vi "PH_gentec_P-Link.set Default Settings.vi"(0 "i ref in":refnum<vi>, 5 "error in":errorcluster) -> (14 "i ref out":refnum<vi>, 19 "error out":errorcluster)   [LabVIEW 2014, in "PH_gentec_P-Link.lvlib"]
doc: "This VI sets Default Settings to wanted Device Settings at own attreibutes. This VI must be placed before the creation of the Proc Events in order to be able to overwrite these later by a Start GOG ..."
uses:
  PH_gentec_P-Link.lvlib
  PH_gentec_M-Link/PH_gentec_M-Link.lvlib
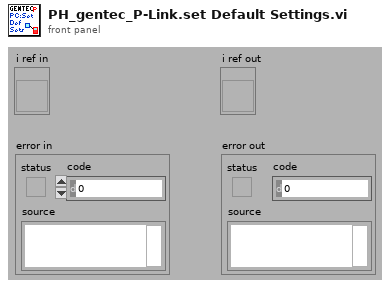
[diagram p1: front panel]
types:
  T1 = typedef "PH_gentec_P-Link.lvlib/PH_gentec_P-Link.i attribute.ctl" = cluster{"GUI References":cluster{"Wanted Head Settings":refnum<vi>, "Current Head Settings":refnum<vi>, "Set Auto Range":refnum<vi>, "Trigger Polarity":refnum<vi>, "Trigger Source":refnum<vi>, "Waveform Averages":refnum<vi>, "Continuous":refnum<vi>, "get one Value":refnum<vi>}, "Wanted Head Settings":T2, "Current Head Settings":T2}
  T2 = typedef "PH_gentec_P-Link.lvlib/PH_gentec_P-Link.Head Settings.ctl" = cluster{"Measurement Mode":T3, "Enable Anticipation":bool, "Set Auto Range":bool, "Block Signal":bool, "Set Head Attenuator":bool, "Enable SSE":bool, "Trigger Polarity":T4, "Trigger Source":T5, "Waveform Averages":T6, "Set Zero":i32, "Current":i32, "Start Data Flow":bool}
  T3 = typedef "gentec-M-Link - Driver.lvlib/gentec-M-Link.Measurement Mode.ctl" = u16
  T4 = typedef "gentec-M-Link - Driver.lvlib/gentec-M-Link.Trigger Polarity.ctl" = u16
  T5 = typedef "gentec-M-Link - Driver.lvlib/gentec-M-Link.Trigger Source.ctl" = u16
  T6 = typedef "gentec-M-Link - Driver.lvlib/gentec-M-Link.Waveform Averages.ctl" = u16
  T7 = typedef "PH_gentec_M-Link.lvlib/PH_gentec_M-Link.Head Settings.ctl" = cluster{"Measurement Mode":T8, "Enable Anticipation":bool, "Set Auto Range":bool, "Block Signal":bool, "Set Head Attenuator":bool, "Range":T9, "Enable SSE":bool, "Trigger Level [%]":dbl, "Trigger Polarity":T10, "Trigger Source":T11, "Waveform Averages":T12, "Wavelength [nm]":u16, "Set Zero":i32, "Current Measurement":i32, "Start Data Flow":bool}
  T8 = typedef "gentec-M-LINK.lvlib/gentec-M-Link.Measurement Mode.ctl" = u16
  T9 = typedef "gentec-M-LINK.lvlib/gentec-M-Link.Range.ctl" = u16
  T10 = typedef "gentec-M-LINK.lvlib/gentec-M-Link.Trigger Polarity.ctl" = u16
  T11 = typedef "gentec-M-LINK.lvlib/gentec-M-Link.Trigger Source.ctl" = u16
  T12 = typedef "gentec-M-LINK.lvlib/gentec-M-Link.Waveform Averages.ctl" = u16
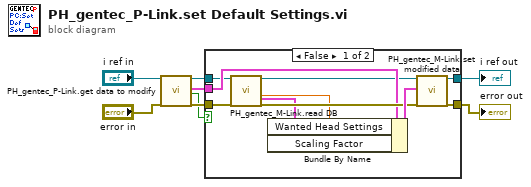
[diagram p0: block diagram]
diagram:
  n1 = call "PH_gentec_P-Link.get data to modify.vi"("i ref in"="i ref in", "error in (no error)"="error in") -> ("i ref out"=w6:refnum<vi>, "i attribute"=w4:T1, "timed out"=w3:bool, "error out"=w5:errorcluster)  [unwired: 14 in]
  n2 = case shown="False" w3 {
    tunnel: [w10 w19] -> w8
    tunnel: [w11 w20] -> w7
    tunnel: w5 -> [w17 w19]
    tunnel: w6 -> [w13 w20]
    tunnel: w4 -> [w15 _]
    frame False {
      n3 = call "PH_gentec_M-Link.read DB.vi"("i ref in"=w13, "error in"=w17) -> ("Default scaling Factor"=w14:dbl, "i ref out"=w12:refnum<vi>, "Default Head Settings"=w9:T7, "error out"=w16:errorcluster)  [unwired: 12 in, 2 out]
      n4 = Bundle By Name(cluster=w15, "Wanted Head Settings"=w9, "Scaling Factor"=w14) -> (w18:T1)
      n5 = call "PH_gentec_M-Link.set modified data.vi"("i ref in"=w12, "i attribute"=w18, "error in (no error)"=w16) -> ("i ref out"=w11:refnum<vi>, "error out"=w10:errorcluster)  [unwired: 15 in]
    }
    frame True {
    }
  }
  "error out" <- w8
  "i ref out" <- w7
